vi "DMA Settings.vi"(6 "Action":T4, 8 "error in (no error)":errorcluster, 10 "DMA Settings":T1={"Number of Channels"=0, "Delacing Scheme"=enum."Interleaved", "Update Rate"=1, "dt"=0.0001, "Mode"=enum."Continuous", "Number of Samples"=10000, "DMA Host Buffer"=5} {"DMA Host Buffer" items=["1 Second"=1, "2 Seconds"=2, "5 Seconds"=5, "10 Seconds"=10]; "dt" format="%#_p"; "Update Rate" items=["1 Hz"=1, "2 Hz"=2, "5 Hz"=5, "10 Hz"=10]}, 11 "Item Ref":T5 format="%.0x") -> (0 "error out":errorcluster, 2 "DMA Settings":T1={"Number of Channels"=1, "Delacing Scheme"=enum."Interleaved", "Update Rate"=1000, "dt"=1000.0, "Mode"=enum."Continuous", "Number of Samples"=0, "DMA Host Buffer"=5} {"DMA Host Buffer" items=["1 Second"=1, "2 Seconds"=2, "5 Seconds"=5, "10 Seconds"=10]; "dt" format="%#_p"; "Update Rate" items=["1 Hz"=1, "2 Hz"=2, "5 Hz"=5, "10 Hz"=10]}, 3 "Item Ref out":T5=18446744073709551615 format="%.0x")   [LabVIEW 2019, in "FPGA Addon Shared.lvlib"]
uses:
  FPGA Addon Shared.lvlib
  Types/DMA Settings.ctl
  Types/Delacing Scheme.ctl
  Types/DMA Acquisition Mode.ctl
  <vilib>/NI VeriStand/Custom Device API/Custom Device Item Ref.ctl
  Types/FG Action.ctl
  Constants.vi
  <vilib>/NI VeriStand/Custom Device API/Get Item Property (U32).vi
  <vilib>/NI VeriStand/Custom Device API/Get Item Property (Double).vi
  <vilib>/NI VeriStand/Custom Device API/Set Item Property (U32).vi
  <vilib>/NI VeriStand/Custom Device API/Set Item Property (Double).vi
  <vilib>/NI VeriStand/Custom Device API/Custom Device API.lvlib
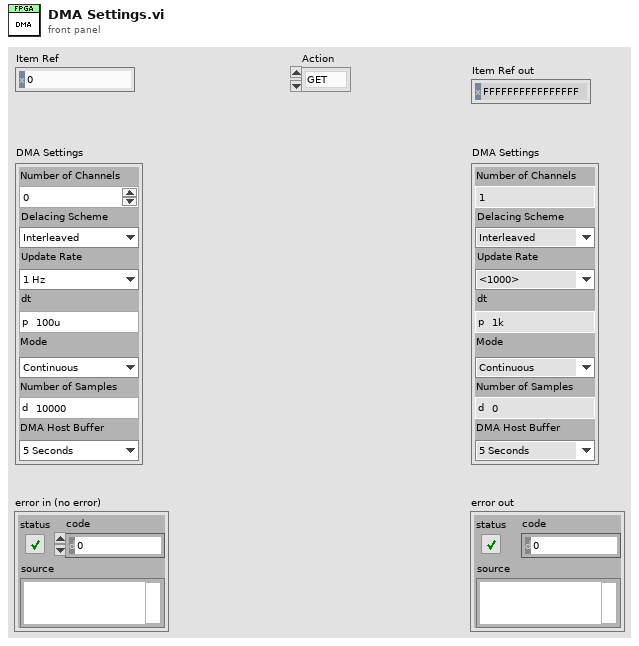
[diagram p1: front panel]
types:
  T1 = typedef "FPGA Addon Shared.lvlib/DMA Settings.ctl" = cluster{"Number of Channels":u8, "Delacing Scheme":T2, "Update Rate":u32, "dt":dbl, "Mode":T3, "Number of Samples":u32, "DMA Host Buffer":u32}
  T2 = typedef "FPGA Addon Shared.lvlib/Delacing Scheme.ctl" = enum8{"Interleaved", "Bitpacked"}
  T3 = typedef "FPGA Addon Shared.lvlib/DMA Acquisition Mode.ctl" = enum8{"Continuous", "Triggered Finite"}
  T4 = typedef "FPGA Addon Shared.lvlib/FG Action.ctl" = enum8{"GET", "SET"}
  T5 = typedef "Custom Device API.lvlib/Custom Device Item Ref.ctl" = u64
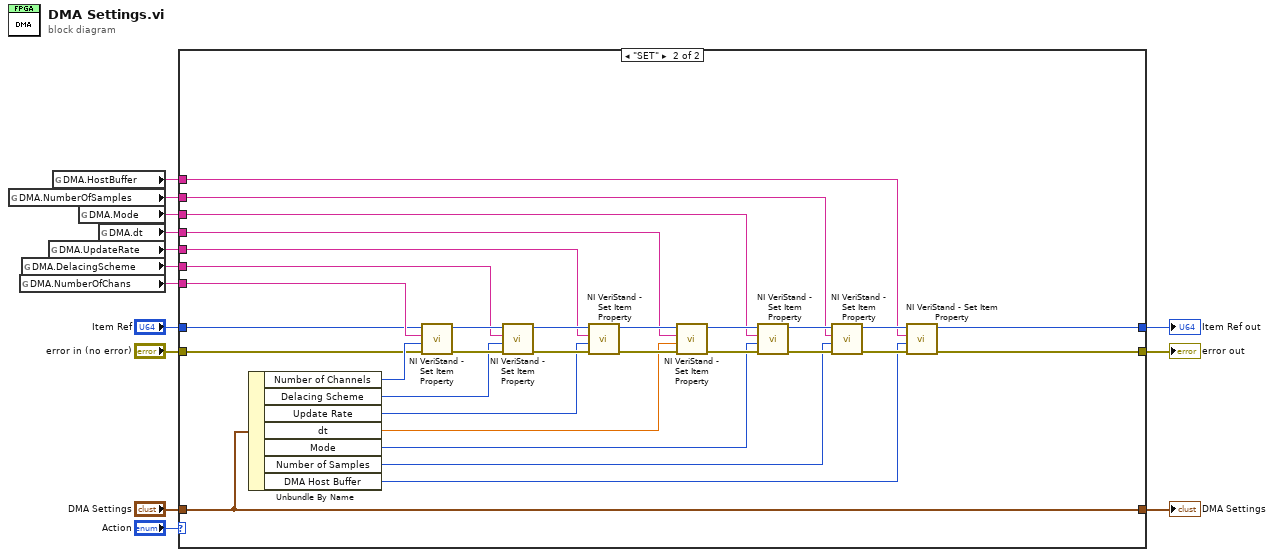
[diagram p0: block diagram]
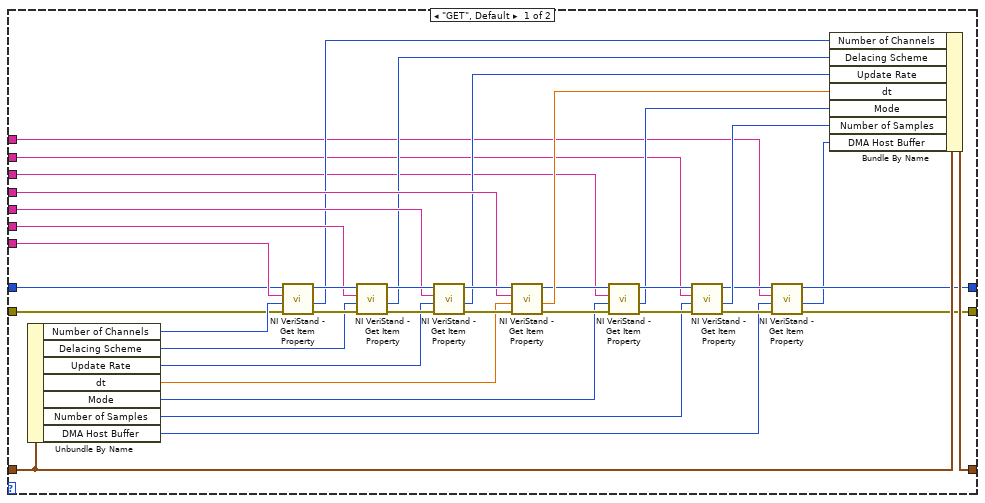
[diagram p2: hidden frame]
diagram:
  n1 = global read "Constants.vi" "DMA.NumberOfSamples"() -> (w2:string)
  n2 = global read "Constants.vi" "DMA.NumberOfChans"() -> (w8:string)
  n3 = global read "Constants.vi" "DMA.DelacingScheme"() -> (w6:string)
  n4 = global read "Constants.vi" "DMA.UpdateRate"() -> (w5:string)
  n5 = global read "Constants.vi" "DMA.HostBuffer"() -> (w1:string)
  n6 = global read "Constants.vi" "DMA.Mode"() -> (w3:string)
  n7 = global read "Constants.vi" "DMA.dt"() -> (w4:string)
  n8 = case shown="\"SET\"" "Action" {
    tunnel: "error in (no error)" -> [w23 w61]
    tunnel: "Item Ref" -> [w22 w60]
    tunnel: "DMA Settings" -> [w35 w70]
    tunnel: [w20 w57] -> w14
    tunnel: [w18 w56] -> w10
    tunnel: [w34 w70] -> w7
    tunnel: w8 -> [w53 w84]
    tunnel: w6 -> [w46 w76]
    tunnel: w5 -> [w45 w75]
    tunnel: w4 -> [w44 w74]
    tunnel: w3 -> [w29 w65]
    tunnel: w2 -> [w25 w64]
    tunnel: w1 -> [w17 w55]
    frame "GET", Default {
      n9 = Unbundle By Name(w35) -> ("Number of Channels"=w40:u8, "Delacing Scheme"=w41:T2, "Update Rate"=w42:u32, "dt"=w43:dbl, "Mode"=w28:T3, "Number of Samples"=w26:u32, "DMA Host Buffer"=w15:u32)
      n10 = call-poly <vilib>:"NI VeriStand - Get Item Property.vi"("error in (no error)"=w23, "Default Value"=w40, "Property Name"=w53, "Item Ref in"=w22) -> ("error out"=w52:errorcluster, "Value"=w39:u32, "Item Ref out"=w47:T5)  [unwired: 4 in, 1 out]
      n11 = call-poly <vilib>:"NI VeriStand - Get Item Property.vi"("error in (no error)"=w52, "Default Value"=w41, "Property Name"=w46, "Item Ref in"=w47) -> ("error out"=w51:errorcluster, "Value"=w38:u32, "Item Ref out"=w48:T5)  [unwired: 4 in, 1 out]
      n12 = call-poly <vilib>:"NI VeriStand - Get Item Property.vi"("error in (no error)"=w51, "Default Value"=w42, "Property Name"=w45, "Item Ref in"=w48) -> ("error out"=w50:errorcluster, "Value"=w37:u32, "Item Ref out"=w49:T5)  [unwired: 4 in, 1 out]
      n13 = call-poly <vilib>:"NI VeriStand - Get Item Property.vi"("error in (no error)"=w50, "Default Value"=w43, "Property Name"=w44, "Item Ref in"=w49) -> ("error out"=w30:errorcluster, "Value"=w36:dbl, "Item Ref out"=w33:T5)  [unwired: 4 in, 1 out]
      n14 = call-poly <vilib>:"NI VeriStand - Get Item Property.vi"("error in (no error)"=w30, "Default Value"=w28, "Property Name"=w29, "Item Ref in"=w33) -> ("error out"=w31:errorcluster, "Value"=w27:u32, "Item Ref out"=w32:T5)  [unwired: 4 in, 1 out]
      n15 = call-poly <vilib>:"NI VeriStand - Get Item Property.vi"("error in (no error)"=w31, "Default Value"=w26, "Property Name"=w25, "Item Ref in"=w32) -> ("error out"=w21:errorcluster, "Value"=w24:u32, "Item Ref out"=w19:T5)  [unwired: 4 in, 1 out]
      n16 = call-poly <vilib>:"NI VeriStand - Get Item Property.vi"("error in (no error)"=w21, "Default Value"=w15, "Property Name"=w17, "Item Ref in"=w19) -> ("error out"=w20:errorcluster, "Value"=w16:u32, "Item Ref out"=w18:T5)  [unwired: 4 in, 1 out]
      n17 = Bundle By Name(cluster=w35, "Number of Channels"=w39, "Delacing Scheme"=w38, "Update Rate"=w37, "dt"=w36, "Mode"=w27, "Number of Samples"=w24, "DMA Host Buffer"=w16) -> (w34:T1)
    }
    frame "SET" {
      n18 = Unbundle By Name(w70) -> ("Number of Channels"=w83:u8, "Delacing Scheme"=w73:T2, "Update Rate"=w72:u32, "dt"=w71:dbl, "Mode"=w63:T3, "Number of Samples"=w62:u32, "DMA Host Buffer"=w54:u32)
      n19 = call-poly <vilib>:"NI VeriStand - Set Item Property.vi"("error in (no error)"=w61, "Value"=w83, "Property Name"=w84, "Item Ref in"=w60) -> ("error out"=w81:errorcluster, "Item Ref out"=w82:T5)  [unwired: 5 in, 1 out]
      n20 = call-poly <vilib>:"NI VeriStand - Set Item Property.vi"("error in (no error)"=w81, "Value"=w73, "Property Name"=w76, "Item Ref in"=w82) -> ("error out"=w77:errorcluster, "Item Ref out"=w80:T5)  [unwired: 5 in, 1 out]
      n21 = call-poly <vilib>:"NI VeriStand - Set Item Property.vi"("error in (no error)"=w77, "Value"=w72, "Property Name"=w75, "Item Ref in"=w80) -> ("error out"=w78:errorcluster, "Item Ref out"=w79:T5)  [unwired: 5 in, 1 out]
      n22 = call-poly <vilib>:"NI VeriStand - Set Item Property.vi"("error in (no error)"=w78, "Value"=w71, "Property Name"=w74, "Item Ref in"=w79) -> ("error out"=w66:errorcluster, "Item Ref out"=w69:T5)  [unwired: 5 in, 1 out]
      n23 = call-poly <vilib>:"NI VeriStand - Set Item Property.vi"("error in (no error)"=w66, "Value"=w63, "Property Name"=w65, "Item Ref in"=w69) -> ("error out"=w67:errorcluster, "Item Ref out"=w68:T5)  [unwired: 5 in, 1 out]
      n24 = call-poly <vilib>:"NI VeriStand - Set Item Property.vi"("error in (no error)"=w67, "Value"=w62, "Property Name"=w64, "Item Ref in"=w68) -> ("error out"=w58:errorcluster, "Item Ref out"=w59:T5)  [unwired: 5 in, 1 out]
      n25 = call-poly <vilib>:"NI VeriStand - Set Item Property.vi"("error in (no error)"=w58, "Value"=w54, "Property Name"=w55, "Item Ref in"=w59) -> ("error out"=w57:errorcluster, "Item Ref out"=w56:T5)  [unwired: 5 in, 1 out]
    }
  }
  "error out" <- w14
  "Item Ref out" <- w10
  "DMA Settings" <- w7
